vi "GetTextPositions.vi"(0 "reference":refnum<class "StateTransitionEdge.lvclass">, 1 "GraphicsRef":refnum<class "Graphics.lvclass">, 5 "error in (no error)":errorcluster) -> (14 "reference out":refnum<class "StateTransitionEdge.lvclass">, 15 "connectionPoints":T1[](array[typedef]) {"y" format="%.2f"; "x" format="%.2f"}, 19 "error out":errorcluster)   [LabVIEW 2012, in "StateTransitionEdge.lvclass"]
doc: "GetTextPositions"
uses:
  <resource>/Framework/Providers/Open_GDS/UML/StateTransitionEdge_class/StateTransitionEdge.lvclass
  <resource>/Framework/Providers/Open_GDS/UML/General/Point/Point Point2D.ctl
  <resource>/Framework/Providers/Open_GDS/UML/Graphics_class/Graphics.lvclass
  <resource>/Framework/Providers/Open_GDS/UML/BentStyle_class/BentStyle.lvclass
  <resource>/Framework/Providers/Open_GDS/UML/ClassRelationshipEdge_class/ClassRelationshipEdge.lvclass
  <resource>/Framework/Providers/Open_GDS/UML/SegmentedLineEdge_class/SegmentedLineEdge.lvclass
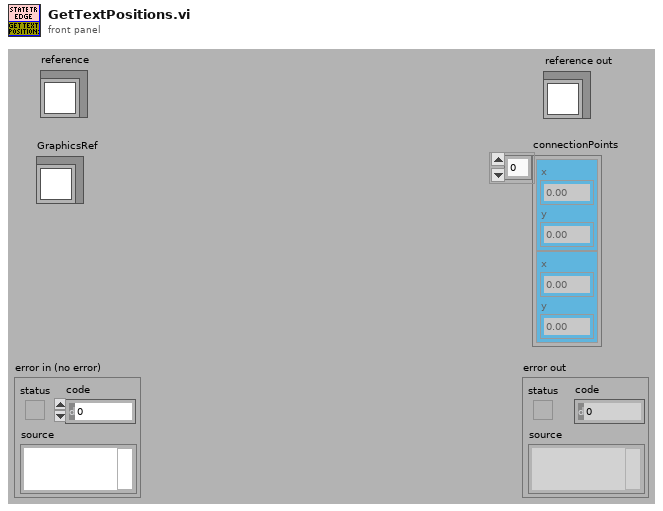
[diagram p1: front panel]
types:
  T1 = typedef "Point Point2D.ctl" = cluster{"x":dbl, "y":dbl}
  T2 = typedef "ClassRelationshipEdge.lvclass/ObjectAttributes.ctl" = cluster{"bentStyleRef":refnum<class "BentStyle.lvclass">, "startConnectionOffset":cluster{"x":i32, "y":i32}, "endConnectionOffset":cluster{"x":i32, "y":i32}, "MidLineOffset":cluster{"x":i32, "y":i32}, "DepClass":T3}
  T3 = typedef "ReversedEngineering_ViDependencyDetailsType.ctl" = cluster{"ThisVIs/Ctls":path[], "Dependent_VIs/Ctls":path[]}
  T4 = typedef "SegmentedLineEdge.lvclass/ObjectAttributes.ctl" = cluster{"lineStyle":refnum<class "LineStyle.lvclass">, "startArrowHead":refnum<class "ArrowHead.lvclass">, "endArrowHead":refnum<class "ArrowHead.lvclass">, "startLabel":string, "midLabel":string, "endLabel":string, "MidLabelOffset":T1, "SplitWire":bool}
  T5 = typedef "BentStyle.lvclass/BentStyleType.ctl" = enum16{"STRAIGHT", "HV", "VH", "HVH", "VHV", "ARC"}
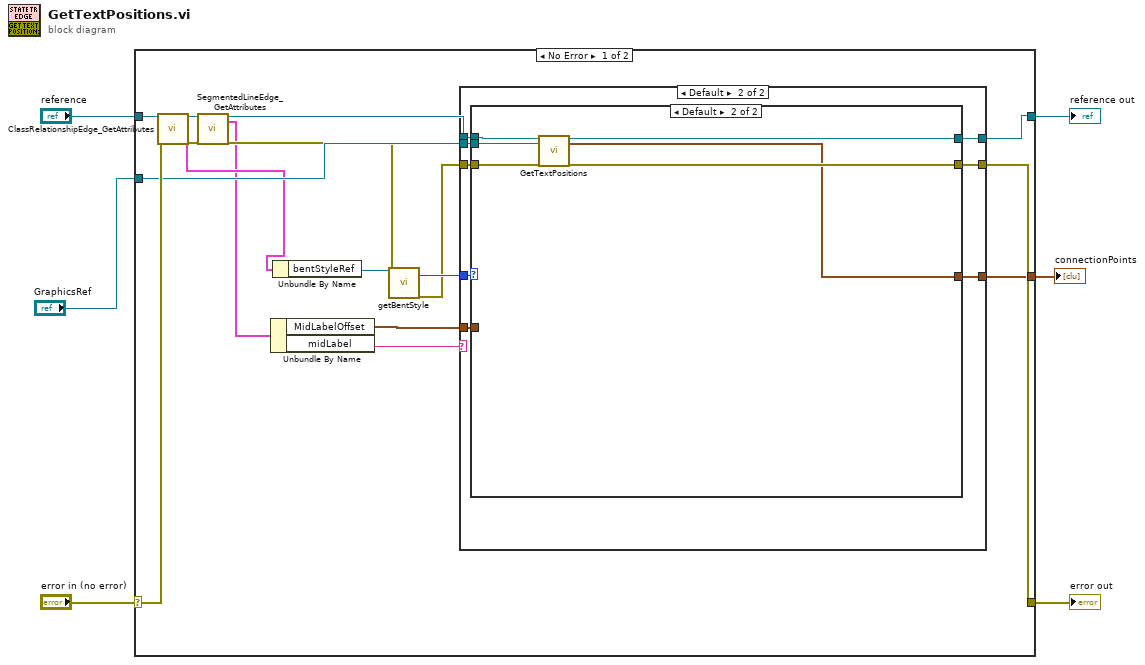
[diagram p0: block diagram]
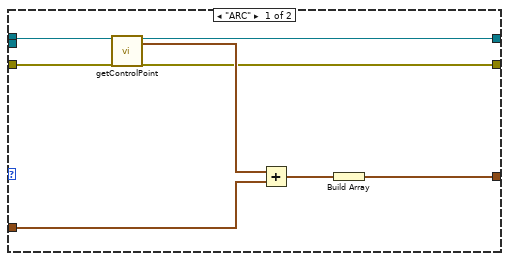
[diagram p3: hidden frame]
diagram:
  n1 = case shown="No Error" "error in (no error)" {
    selector: "error in (no error)" -> [w23 w48]
    tunnel: "reference" -> [w22 w49]
    tunnel: [w17 w48] -> w4
    tunnel: [w16 w49] -> w3
    tunnel: [w15 _] -> w2
    tunnel: "GraphicsRef" -> [w13 _]
    frame No Error {
      n2 = call <resource>:"ClassRelationshipEdge_GetAttributes.vi"("reference in"=w22, "error in (no error)"=w23) -> ("reference out"=w11:refnum<class "StateTransitionEdge.lvclass">, "Data"=w12:T2, "error out"=w10:errorcluster)  [unwired: 14 in, 1 out]
      n3 = call <resource>:"SegmentedLineEdge_GetAttributes.vi"("reference in"=w11, "error in (no error)"=w10) -> ("reference out"=w8:refnum<class "StateTransitionEdge.lvclass">, "Data"=w7:T4, "error out"=w9:errorcluster)  [unwired: 14 in, 1 out]
      n4 = Unbundle By Name(w7) -> ("MidLabelOffset"=w18:T1, "midLabel"=w14:string)
      n5 = Unbundle By Name(w12) -> ("bentStyleRef"=w21:refnum<class "BentStyle.lvclass">)
      n6 = call-dynamic "getBentStyle.vi"("reference"=w21, "error in (no error)"=w9) -> ("bentStyle"=w20:T5, "error out"=w19:errorcluster)  [unwired: 15 in, 1 out]
      n7 = case shown="Default" w14 {
        tunnel: w20 -> [_ w33]
        tunnel: w19 -> [w25 w32]
        tunnel: w18 -> [_ w31]
        tunnel: w8 -> [w24 w30]
        tunnel: [w25 w29] -> w17
        tunnel: [w24 w28] -> w16
        tunnel: [_ w27] -> w15
        tunnel: w13 -> [_ w26]
        frame "" {
        }
        frame Default {
          n8 = case shown="Default" w33 {
            tunnel: w30 -> [w37 w47]
            tunnel: w32 -> [w36 w46]
            tunnel: [w39 w44] -> w29
            tunnel: [w38 w45] -> w28
            tunnel: w31 -> [w34 _]
            tunnel: [w40 w43] -> w27
            tunnel: w26 -> [_ w42]
            frame "ARC" {
              n9 = call <resource>:"getControlPoint.vi"("reference"=w37, "error in (no error)"=w36) -> ("reference out"=w38:refnum<class "StateTransitionEdge.lvclass">, "point"=w41:T1, "error out"=w39:errorcluster)  [unwired: 15 out]
              n10 = Add(x=w41, y=w34) -> (x+y=w35:T1)
              n11 = Build Array(w35) -> (w40:T1[])
            }
            frame Default {
              n12 = call-parent "GetTextPositions.vi"("reference"=w47, "GraphicsRef"=w42, "error in (no error)"=w46) -> ("reference out"=w45:refnum<class "StateTransitionEdge.lvclass">, "connectionPoints"=w43:T1[], "error out"=w44:errorcluster)  [unwired: 14 in]
            }
          }
        }
      }
    }
    frame Error {
    }
  }
  "reference out" <- w3
  "error out" <- w4
  "connectionPoints" <- w2
